vi "状态查询.vi"() -> ()   [LabVIEW 2016, in "流量计集成.lvlib" / "LSS-100X流量计.lvlib"]
uses:
  <vilib>/Plasmionique/MB Master/MB_Master_Serial/MB_Master_Serial.lvclass
  C:/Program Files (x86)/National Instruments/LabVIEW 2016/vi.lib/Plasmionique/MB Master/MB_Master/MB_Master.lvclass
  <vilib>/Plasmionique/MB Master/MB Master.lvlib
panel:
  out "错误代码":u16
  in  "站号":u8=1
  in  "关闭":bool
  in  "刷新按钮":bool
  out "下游信号强度":u16
  out "上游信号强度":u16
  out "信号质量":u16
  out "错误信息":string
  out "正累计流量":u32
  out "测量流体声速":sgl
  out "流体速度":sgl
  out "瞬时热流量":sgl
  out "瞬时流量":sgl
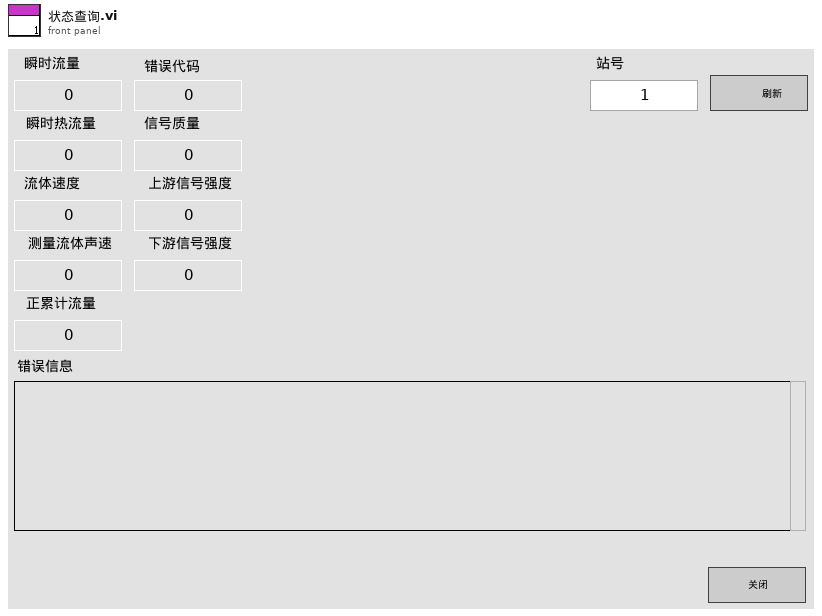
[diagram p1: front panel]
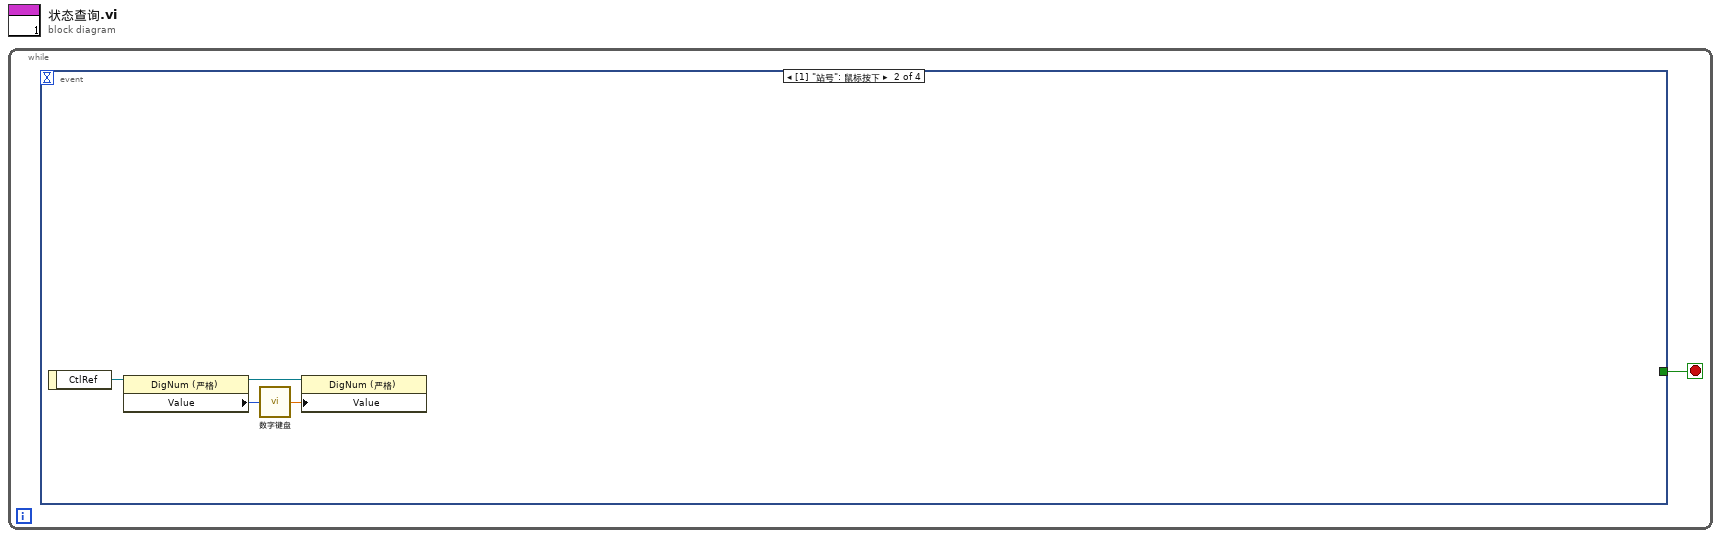
[diagram p0: block diagram]
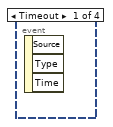
[diagram p2: hidden frame]
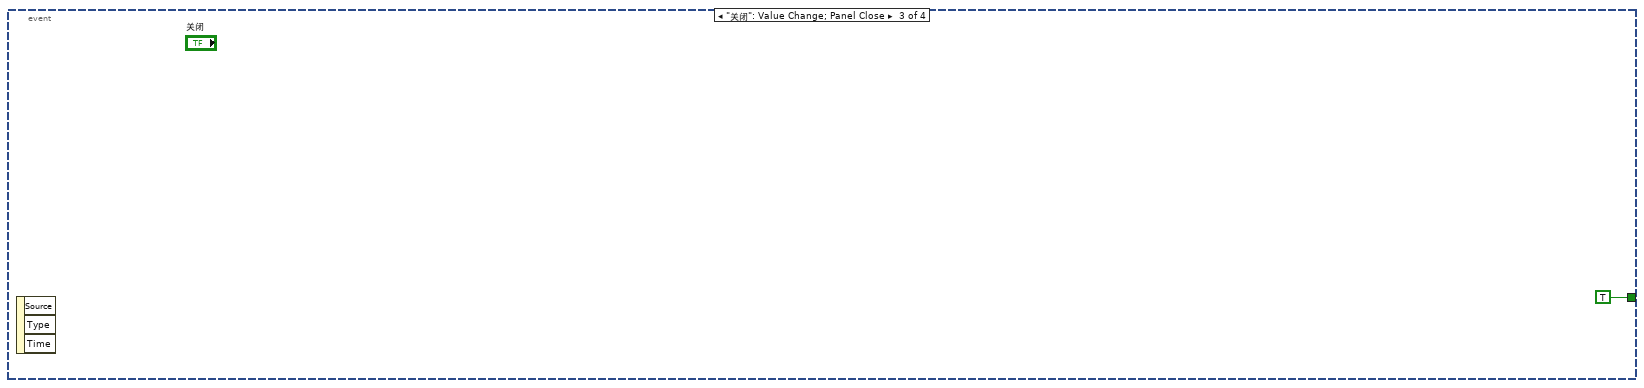
[diagram p3: hidden frame]
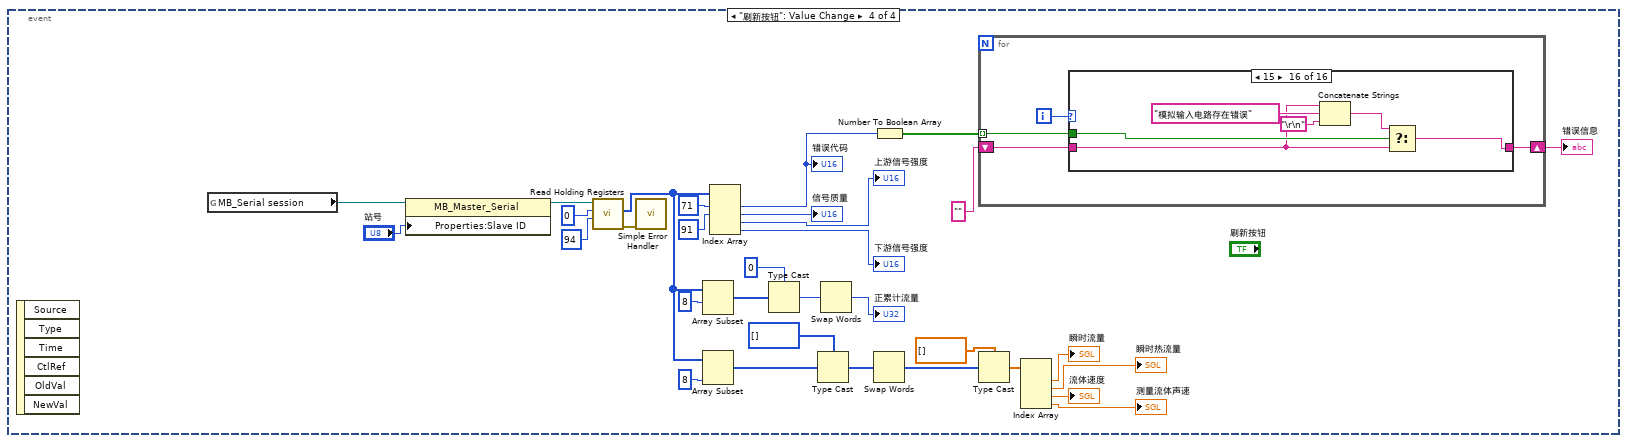
[diagram p4: hidden frame]
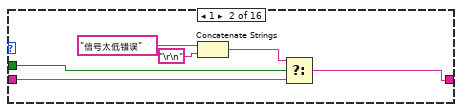
[diagram p6: hidden frame]
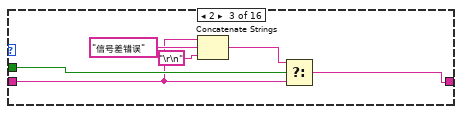
[diagram p7: hidden frame]
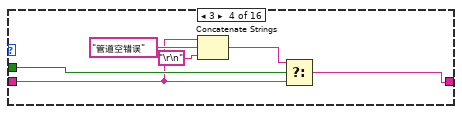
[diagram p8: hidden frame]
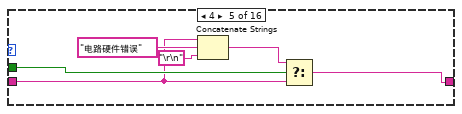
[diagram p9: hidden frame]
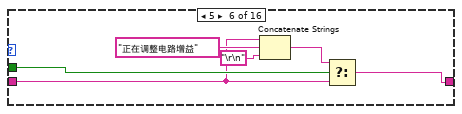
[diagram p10: hidden frame]
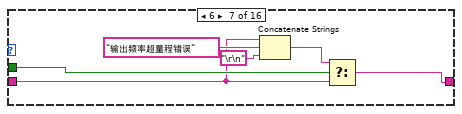
[diagram p11: hidden frame]
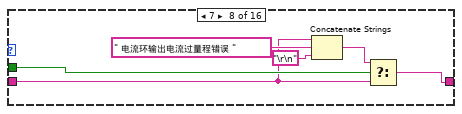
[diagram p12: hidden frame]
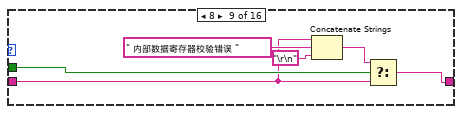
[diagram p13: hidden frame]
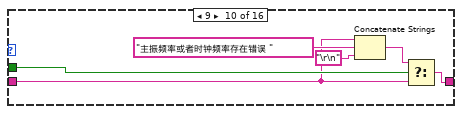
[diagram p14: hidden frame]
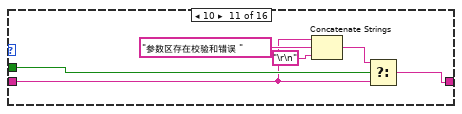
[diagram p15: hidden frame]
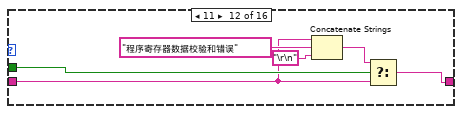
[diagram p16: hidden frame]
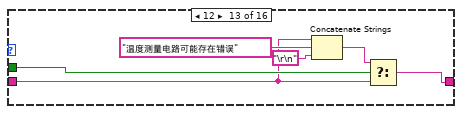
[diagram p17: hidden frame]
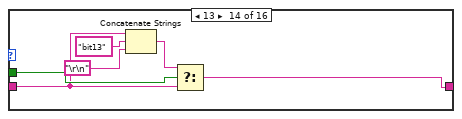
[diagram p18: hidden frame]
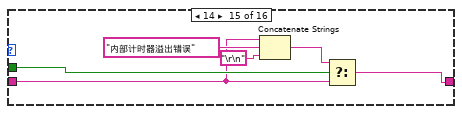
[diagram p19: hidden frame]
diagram:
  n1 = while {
    stop <- w1 stop-if-true
    n2 = event shown="[1] \"站号\": 鼠标按下" {
      selector: _ -> [_ _ _ _]
      dyn-events: _ -> [_ _ _ _]
      timeout: _ -> [_ _ _ _]
      tunnel: [_ _ TRUE _] -> w1
      event Timeout {
        n3 = event-data() -> ()  [unwired: 1 in, 3 out]
      }
      event "站号": Mouse Down {
        n4 = event-data() -> ("CtlRef"=w5:refnum<vi>)  [unwired: 1 in]
        n5 = property class="DigNum (严格)"(reference=w5) -> (reference out=w3:refnum<vi>, "Value"=w4:u8)  [unwired: 1 in, 1 out]
        n6 = call "数字键盘.vi"("OldNumber"=w4) -> ("NewNumber"=w2:dbl)
        n7 = property class="DigNum (严格)"(reference=w3, "Value"=w2) -> ()  [unwired: 1 in, 2 out]
      }
      event "关闭": Value Change; Panel Close {
        n8 = event-data() -> ()  [unwired: 1 in, 3 out]
      }
      event "刷新按钮": Value Change {
        n9 = event-data() -> ()  [unwired: 1 in, 6 out]
        n10 = global read "流量计全局变量.vi" "MB_Serial session"() -> (w12:refnum<class "MB_Master_Serial.lvclass">)
        n11 = property class="MB_Master_Serial"(reference=w12, "Properties:Slave ID"="站号") -> (reference out=w10:refnum<class "MB_Master_Serial.lvclass">)  [unwired: 1 in, 1 out]
        n12 = call <vilib>:"Read Holding Registers.vi"("quantity"=u16 94 ("starting address"), "starting address"=u16 0, "MB session in"=w10) -> ("error out"=w7:errorcluster, "Registers"=w29:u16[])  [unwired: 6 in, 1 out]
        n13 = call <vilib>:"Simple Error Handler.vi"("error in (no error)"=w7) -> ()  [unwired: 4 in, 5 out]
        n14 = Array Subset(array=w29, index=8 ("索引")) -> (w26:u16[])  [unwired: 1 in]
        n15 = Array Subset(array=w29, length=8 ("长度")) -> (w18:u16[])  [unwired: 1 in]
        n16 = Index Array(array=w29, index #1=71 ("索引"), index #2=91 ("索引")) -> (element #1=w35:u16, element #2=→"信号质量":u16, element #3=→"上游信号强度":u16, element #4=→"下游信号强度":u16)  [unwired: 2 in]
        "错误代码" <- w35
        n17 = Type Cast(type=u32 0 ("x/y"), x=w26) -> (*(type *) &x=w27:u32)
        n18 = Type Cast(type=u32[] [], x=w18) -> (*(type *) &x=w15:u32[])
        n19 = Swap Words(1:w27) -> (0:→"正累计流量":u32)
        n20 = Swap Words(1:w15) -> (0:w16:u32[])
        n21 = Number To Boolean Array(number=w35) -> (Boolean array=w36:bool[])
        n22 = for {
          tunnel: w36 -> [w41] mode=indexing
          shift-right: [w40] -> w38
          shift-left: "" -> [w39]
          i -> [w42]
          n23 = case shown="15" w42 {
            tunnel: w41 -> [_ w49 w55 w61 w67 w73 w79 w85 w91 w97 w103 w109 w115 w121 w127 w133]
            tunnel: [w43 w48 w54 w60 w66 w72 w78 w84 w90 w96 w102 w108 w114 w120 w126 w132] -> w40
            tunnel: w39 -> [w43 w47 w50 w56 w62 w68 w74 w80 w86 w92 w98 w104 w110 w116 w122 w128]
            frame Default {
            }
            frame 1 {
              n24 = Concatenate Strings("信号太低错误", "\r\n") -> (w44:string)
              n25 = Select(t=w44, s=w49, f=w47) -> (s? t:f=w48:string)
            }
            frame 2 {
              n26 = Concatenate Strings(w50, "信号差错误", "\r\n") -> (w51:string)
              n27 = Select(t=w51, s=w55, f=w50) -> (s? t:f=w54:string)
            }
            frame 3 {
              n28 = Concatenate Strings(w56, "管道空错误", "\r\n") -> (w57:string)
              n29 = Select(t=w57, s=w61, f=w56) -> (s? t:f=w60:string)
            }
            frame 4 {
              n30 = Concatenate Strings(w62, "电路硬件错误", "\r\n") -> (w63:string)
              n31 = Select(t=w63, s=w67, f=w62) -> (s? t:f=w66:string)
            }
            frame 5 {
              n32 = Concatenate Strings(w68, "正在调整电路增益", "\r\n") -> (w69:string)
              n33 = Select(t=w69, s=w73, f=w68) -> (s? t:f=w72:string)
            }
            frame 6 {
              n34 = Concatenate Strings(w74, "输出频率超量程错误", "\r\n") -> (w75:string)
              n35 = Select(t=w75, s=w79, f=w74) -> (s? t:f=w78:string)
            }
            frame 7 {
              n36 = Concatenate Strings(w80, " 电流环输出电流过量程错误 ", "\r\n") -> (w81:string)
              n37 = Select(t=w81, s=w85, f=w80) -> (s? t:f=w84:string)
            }
            frame 8 {
              n38 = Concatenate Strings(w86, " 内部数据寄存器校验错误 ", "\r\n") -> (w87:string)
              n39 = Select(t=w87, s=w91, f=w86) -> (s? t:f=w90:string)
            }
            frame 9 {
              n40 = Concatenate Strings(w92, "主振频率或者时钟频率存在错误 ", "\r\n") -> (w93:string)
              n41 = Select(t=w93, s=w97, f=w92) -> (s? t:f=w96:string)
            }
            frame 10 {
              n42 = Concatenate Strings(w98, "参数区存在校验和错误 ", "\r\n") -> (w99:string)
              n43 = Select(t=w99, s=w103, f=w98) -> (s? t:f=w102:string)
            }
            frame 11 {
              n44 = Concatenate Strings(w104, "程序寄存器数据校验和错误", "\r\n") -> (w105:string)
              n45 = Select(t=w105, s=w109, f=w104) -> (s? t:f=w108:string)
            }
            frame 12 {
              n46 = Concatenate Strings(w110, "温度测量电路可能存在错误", "\r\n") -> (w111:string)
              n47 = Select(t=w111, s=w115, f=w110) -> (s? t:f=w114:string)
            }
            frame 13 {
              n48 = Concatenate Strings(w116, "bit13", "\r\n") -> (w117:string)
              n49 = Select(t=w117, s=w121, f=w116) -> (s? t:f=w120:string)
            }
            frame 14 {
              n50 = Concatenate Strings(w122, "内部计时器溢出错误", "\r\n") -> (w123:string)
              n51 = Select(t=w123, s=w127, f=w122) -> (s? t:f=w126:string)
            }
            frame 15 {
              n52 = Concatenate Strings(w128, "模拟输入电路存在错误", "\r\n") -> (w129:string)
              n53 = Select(t=w129, s=w133, f=w128) -> (s? t:f=w132:string)
            }
          }
        }
        "错误信息" <- w38
        n54 = Type Cast(type=sgl[] [], x=w16) -> (*(type *) &x=w17:sgl[])
        n55 = Index Array(array=w17) -> (element #1=→"瞬时流量":sgl, element #2=→"瞬时热流量":sgl, element #3=→"流体速度":sgl, element #4=→"测量流体声速":sgl)  [unwired: 4 in]
      }
    }
  }
